vi "TimerGen.vi"(8 "error In":errorcluster, 9 "Interval(s)":dbl=60.0 caption="Intervalle\nd'acq. (s)" min=0.1 step=0.1 format="%#.1f", 10 "TimeLeftRef":refnum<vi>, 11 "UpdateRef":refnum<vi>) -> (0 "error out":errorcluster, 1 "TempsRest":dbl caption="Temps Restant" format="%<%H:%M:%S%1u>t", 2 "Delta(ms)":u32, 3 "FinalTime(ms)":u32)   [LabVIEW 2019]
uses:
  <userlib>/GenProg/ReadbyWeakRefBool.vi
panel:
  out "InitTime(ms)":u32
  in  "MiseAJour":bool
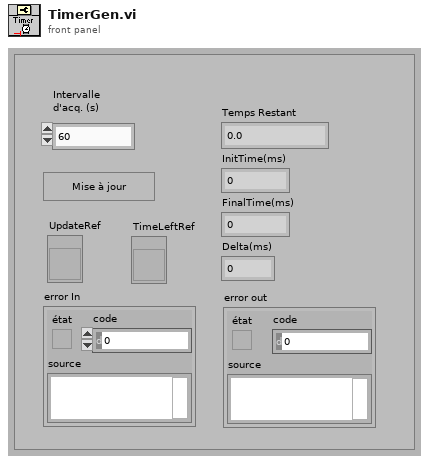
[diagram p1: front panel]
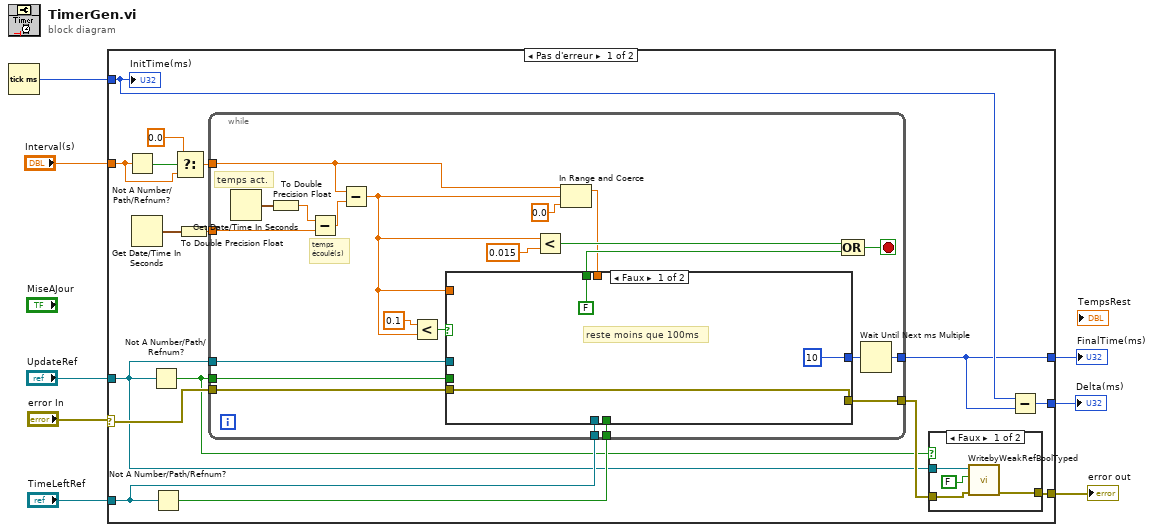
[diagram p0: block diagram]
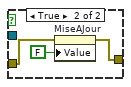
[diagram p2: hidden frame]
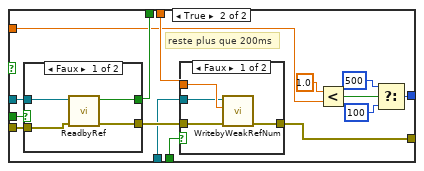
[diagram p3: hidden frame]
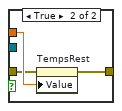
[diagram p4: hidden frame]
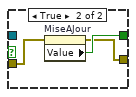
[diagram p5: hidden frame]
diagram:
  n1 = Tick Count (ms)() -> (millisecond timer value=w3:u32)
  n2 = case shown="Pas d'erreur" "error In" {
    selector: "error In" -> [w22 w86]
    tunnel: "Interval(s)" -> [w10 _]
    tunnel: "UpdateRef" -> [w17 _]
    tunnel: [w16 w86] -> w5
    tunnel: [w13 _] -> w4
    tunnel: w3 -> [w15 _]
    tunnel: "TimeLeftRef" -> [w19 _]
    tunnel: [w14 _] -> w1
    frame No Error {
      n3 = Not A Number/Path/Refnum?(number/path/refnum=w10) -> (NaN/Path/Refnum?=w12:bool)
      n4 = Get Date/Time In Seconds() -> (seconds since 1Jan1904=w24:timestamp)
      n5 = Not A Number/Path/Refnum?(number/path/refnum=w17) -> (NaN/Path/Refnum?=w18:bool)
      n6 = Not A Number/Path/Refnum?(number/path/refnum=w19) -> (NaN/Path/Refnum?=w20:bool)
      n7 = Select(t=0.0 ("cas vrai"), s=w12, f=w10) -> (s? t:f=w9:dbl)
      n8 = To Double Precision Float(number=w24) -> (double precision float=w23:dbl)
      n9 = while {
        tunnel: w23 -> [w48]
        tunnel: w18 -> [w43]
        tunnel: w17 -> [w42]
        tunnel: w22 -> [w41]
        tunnel: [w40] -> w13
        tunnel: [w35] -> w21
        tunnel: w20 -> [w38]
        tunnel: w19 -> [w37]
        tunnel: w9 -> [w32]
        stop <- w50 stop-if-true
        # "temps\nécoulé(s)"
        # "temps act."
        n10 = Get Date/Time In Seconds() -> (seconds since 1Jan1904=w53:timestamp)
        n11 = To Double Precision Float(number=w53) -> (double precision float=w52:dbl)
        n12 = Subtract(x=w52, y=w48) -> (x-y=w51:dbl)
        n13 = Subtract(x=w32, y=w51) -> (x-y=w33:dbl)
        n14 = Less?(x=0.1, y=w33) -> (x < y?=w34:bool)
        n15 = Less?(x=w33, y=0.015) -> (x < y?=w45:bool)
        n16 = In Range and Coerce(upper limit=w32, x=w33, lower limit=0.0) -> (coerced(x)=w39:dbl)  [unwired: 1 out]
        n17 = case shown="Faux" w34 {
          tunnel: [FALSE ("Value") w71] -> w44
          tunnel: w43 -> [_ w70]
          tunnel: w42 -> [_ w69]
          tunnel: w41 -> [w56 w68]
          tunnel: w39 -> [_ w67]
          tunnel: w38 -> [_ w65]
          tunnel: w37 -> [_ w64]
          tunnel: [u32 10 ("cas faux") w59] -> w36
          tunnel: [w56 w57] -> w35
          tunnel: w33 -> [_ w58]
          frame False {
            # "reste moins que 100ms"
          }
          frame True {
            # "reste plus que 200ms"
            n18 = case shown="Faux" w70 {
              tunnel: [w82 w85] -> w71
              tunnel: w69 -> [w81 _]
              tunnel: w68 -> [w80 w84]
              tunnel: [w79 w83] -> w66
              frame False {
                n19 = call-poly <userlib>:"ReadbyRef.vi"("error in"=w80, "Control Ref"=w81) -> ("error out"=w79:errorcluster, "Valeur"=w82:bool)  [unwired: 8 in]
              }
              frame True {
                n20 = property on="MiseAJour" class="Bool (strict)"(error in=w84) -> (error out=w83:errorcluster, "Value"=w85:bool)  [unwired: 1 in, 1 out]
              }
            }
            n21 = case shown="Faux" w65 {
              tunnel: w67 -> [w75 w77]
              tunnel: [w74 w78] -> w57
              tunnel: w66 -> [w73 w76]
              tunnel: w64 -> [w72 _]
              frame False {
                n22 = call <userlib>:"WritebyWeakRefNum.vi"("error in"=w73, "Valeur"=w75, "Control Ref"=w72) -> ("error out"=w74:errorcluster)  [unwired: 8 in]
              }
              frame True {
                n23 = property on="TempsRest" class="NumNb (strict)"(error in=w76, "Value"=w77) -> (error out=w78:errorcluster)  [unwired: 1 in, 1 out]
              }
            }
            n24 = Less?(x=1.0, y=w58) -> (x < y?=w62:bool)
            n25 = Select(t=u32 500, s=w62, f=u32 100 ("cas faux")) -> (s? t:f=w59:u32)
          }
        }
        n26 = Compound Arithmetic op=OR(w45, w44) -> (w50:bool)
        n27 = Wait Until Next ms Multiple(millisecond multiple=w36) -> (millisecond timer value=w40:u32)
      }
      n28 = case shown="Faux" w18 {
        tunnel: w21 -> [w28 w31]
        tunnel: [w27 w30] -> w16
        tunnel: w17 -> [w25 _]
        frame False {
          n29 = call <userlib>:"WritebyWeakRefBoolTyped.vi"("error in"=w28, "Valeur"=FALSE, "Control Ref"=w25) -> ("error out"=w27:errorcluster)  [unwired: 8 in]
        }
        frame True {
          n30 = property on="MiseAJour" class="Bool (strict)"(error in=w31, "Value"=FALSE ("MiseAJour")) -> (error out=w30:errorcluster)  [unwired: 1 in, 1 out]
        }
      }
      n31 = Subtract(x=w15, y=w13) -> (x-y=w14:u32)
      "InitTime(ms)" <- w15
    }
    frame Error {
    }
  }
  "error out" <- w5
  "FinalTime(ms)" <- w4
  "Delta(ms)" <- w1
